vi "TEST_ASIC_COMPLETE_(ALL).vi"() -> ()   [LabVIEW 2012]
uses:
  <vilib>/Utility/NIReport.llb/NI_report.lvclass
  <vilib>/Utility/NIReport.llb/HTML/NI_HTML.lvclass
panel:
  in  "Majority Test":bool=TRUE
  in  "SumNAdder\n      Test":bool=TRUE
  in  "Sum Test":bool=TRUE
  in  "Instrument VISA in":T1={"AWG VISA"="AgilentGenerator1", "Oscilloscope  VISA "="AgilentOsciloscope", "Integration Board IP"="172.16.7.43", "connection ID"=refnum, "report out"=refnum, "report file path"=path "C:/Users/omartinez/Desktop/L0nL1_Results"}
  out "Instrument VISA out":T1={"AWG VISA"="generadorpulsos", "Oscilloscope  VISA "="Oscilloscope", "Integration Board IP"="172.16.7.43", "connection ID"=refnum, "report out"=refnum, "report file path"=path "C:/Documents and Settings/CTA_LAB01/Desktop/L0_Asic/L0 Asic Test Data"}
  out "error out":errorcluster
  in  "error in":errorcluster
  # "----------->>>>  IN CASE OF MALFUNCTION OR DOUBT CALL: 4164 and/or 2711\n                                    OR EMAIL: omartinez@ifae.es   and/or   rlopez@ifae.es   <<<<<<-----------------"
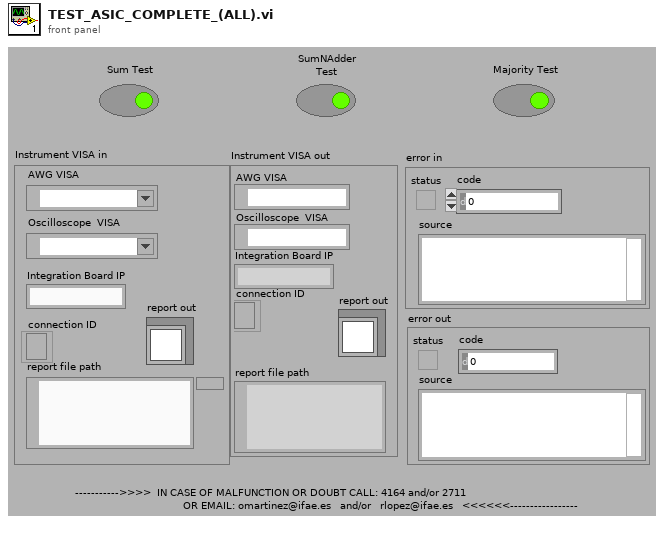
[diagram p1: front panel]
types:
  T1 = cluster{"AWG VISA":refnum<visa-resource-name>, "Oscilloscope  VISA ":refnum<visa-resource-name>, "Integration Board IP":string, "connection ID":refnum<k5>, "report out":refnum<class "NI_report.lvclass">, "report file path":path}
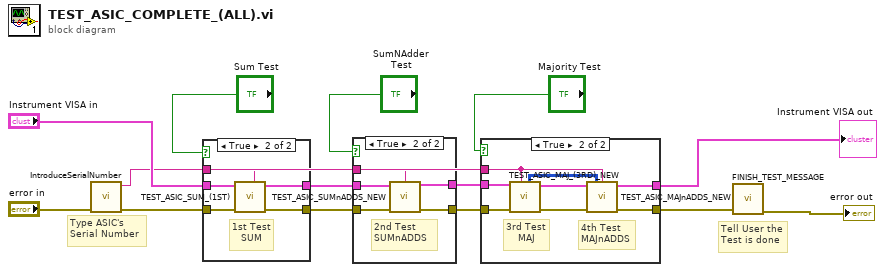
[diagram p0: block diagram]
diagram:
  # "Tell User the\nTest is done"
  # "Type ASIC's\nSerial Number"
  n1 = call "IntroduceSerialNumber.vi"("error in"="error in") -> ("error out"=w7:errorcluster, "Serial Number"=w6:string)  [unwired: 9 in]
  n2 = case shown="True" "Sum Test" {
    tunnel: [w16 w21] -> w14
    tunnel: [w15 w20] -> w11
    tunnel: "Instrument VISA in" -> [w16 w19]
    tunnel: w7 -> [w15 w18]
    tunnel: w6 -> [_ w17]
    frame False {
    }
    frame True {
      # "1st Test\n   SUM"
      n3 = call "TEST_ASIC_SUM_(1ST).vi"("Serial number"=w17, "error in"=w18, "Instrument VISA in"=w19) -> ("error out"=w20:errorcluster, "Instrument VISA out"=w21:T1)  [unwired: 7 in]
    }
  }
  n4 = case shown="True" "SumNAdder\n      Test" {
    tunnel: w14 -> [w23 w25]
    tunnel: [w23 w26] -> w13
    tunnel: w11 -> [w22 w28]
    tunnel: [w22 w27] -> w10
    tunnel: w6 -> [_ w24]
    frame False {
    }
    frame True {
      # "2nd Test\nSUMnADDS"
      n5 = call "TEST_ASIC_SUMnADDS_NEW.vi"("Instrument VISA in"=w25, "Serial number"=w24, "error in"=w28) -> ("Instrument VISA out"=w26:T1, "error out"=w27:errorcluster)  [unwired: 11 in]
    }
  }
  n6 = case shown="True" "Majority Test" {
    tunnel: w13 -> [w30 w38]
    tunnel: [w30 w36] -> w12
    tunnel: w10 -> [w29 w37]
    tunnel: [w29 w35] -> w1
    tunnel: w6 -> [_ w32]
    frame False {
    }
    frame True {
      # "4th Test\nMAJnADDS"
      # "3rd Test\n    MAJ"
      n7 = call "TEST_ASIC_MAJ_(3RD)_NEW.vi"("Serial number"=w32, "error in"=w37, "Instrument VISA in"=w38) -> ("error out"=w33:errorcluster, "Instrument VISA out"=w34:T1, "ThresholdOut"=w31:i32[][])  [unwired: 6 in]
      n8 = call "TEST_ASIC_MAJnADDS_NEW.vi"("Instrument VISA in"=w34, "threshold"=w31, "Serial number"=w32, "error in"=w33) -> ("Instrument VISA out"=w36:T1, "error out"=w35:errorcluster)  [unwired: 10 in]
    }
  }
  "Instrument VISA out" <- w12
  n9 = call "FINISH_TEST_MESSAGE.vi"("error in"=w1) -> ("error out"=→"error out":errorcluster)  [unwired: 10 in]
